vi "capex chambers.vi"(11 "stop":bool) -> ()   [LabVIEW 2013]
panel:
  in  "Minutes displayed":dbl=60.0
  out "Sensor 3 Temperature":waveform(dbl)(graph)={"t0"=timestamp(3552338969.221673 s since 1904-01-01), "dt"=0.001, "Y"=[19.008294294897723], "attributes"=variant("NI_ChannelName"=variant(string "Temp3"), "NI_UnitDescription"=variant(string "Amps"))}
  out "Sensor 3 Humidity":waveform(dbl)(graph)={"t0"=timestamp(3552338969.221658 s since 1904-01-01), "dt"=0.001, "Y"=[61.16415083954544], "attributes"=variant("NI_ChannelName"=variant(string "Humidity3"), "NI_UnitDescription"=variant(string "Amps"))}
  out "Sensor 2 Temperature":waveform(dbl)(graph)={"t0"=timestamp(3552338969.221643 s since 1904-01-01), "dt"=0.001, "Y"=[17.601047768518942], "attributes"=variant("NI_ChannelName"=variant(string "Temp2"), "NI_UnitDescription"=variant(string "Amps"))}
  out "Sensor 2 Humidity":waveform(dbl)(graph)={"t0"=timestamp(3552338969.221613 s since 1904-01-01), "dt"=0.001, "Y"=[70.37875059333966], "attributes"=variant("NI_ChannelName"=variant(string "Humidity2"), "NI_UnitDescription"=variant(string "Amps"))}
  out "Sensor 1 Temperature":waveform(dbl)(graph)={"t0"=timestamp(3552338969.221628 s since 1904-01-01), "dt"=0.001, "Y"=[17.486537818762628], "attributes"=variant("NI_ChannelName"=variant(string "Temp1"), "NI_UnitDescription"=variant(string "Amps"))}
  out "Sensor 1 Humidity":waveform(dbl)(graph)={"t0"=timestamp(3552338969.221598 s since 1904-01-01), "dt"=0.001, "Y"=[66.037122005], "attributes"=variant("NI_ChannelName"=variant(string "Humidity1"), "NI_UnitDescription"=variant(string "Amps"))}
  # "Chamber Temperatures and Humidities as reported by Omega boxes on walls"
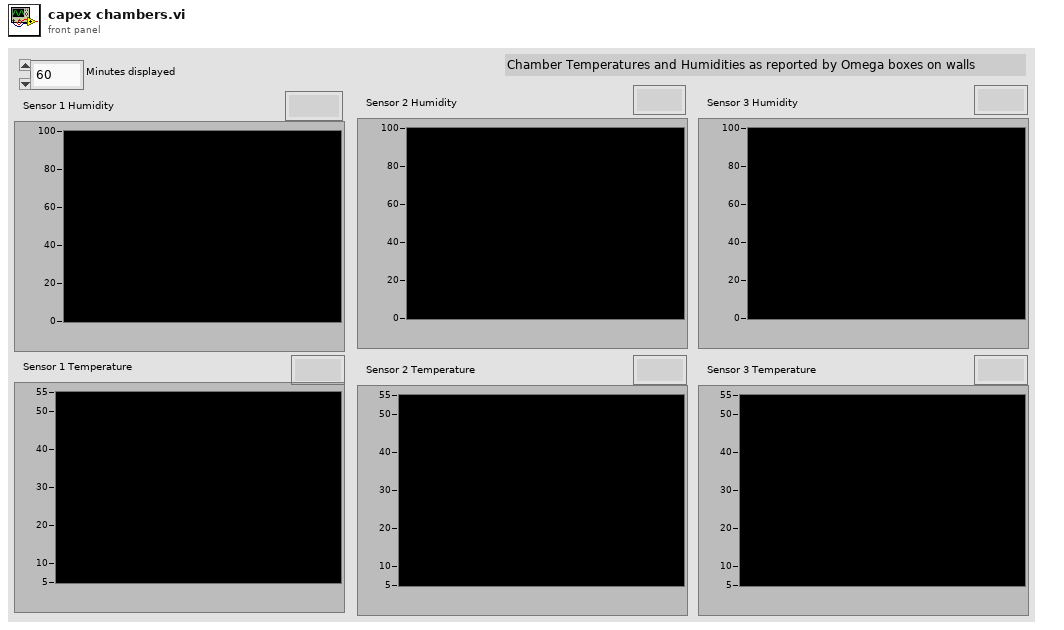
[diagram p1: front panel]
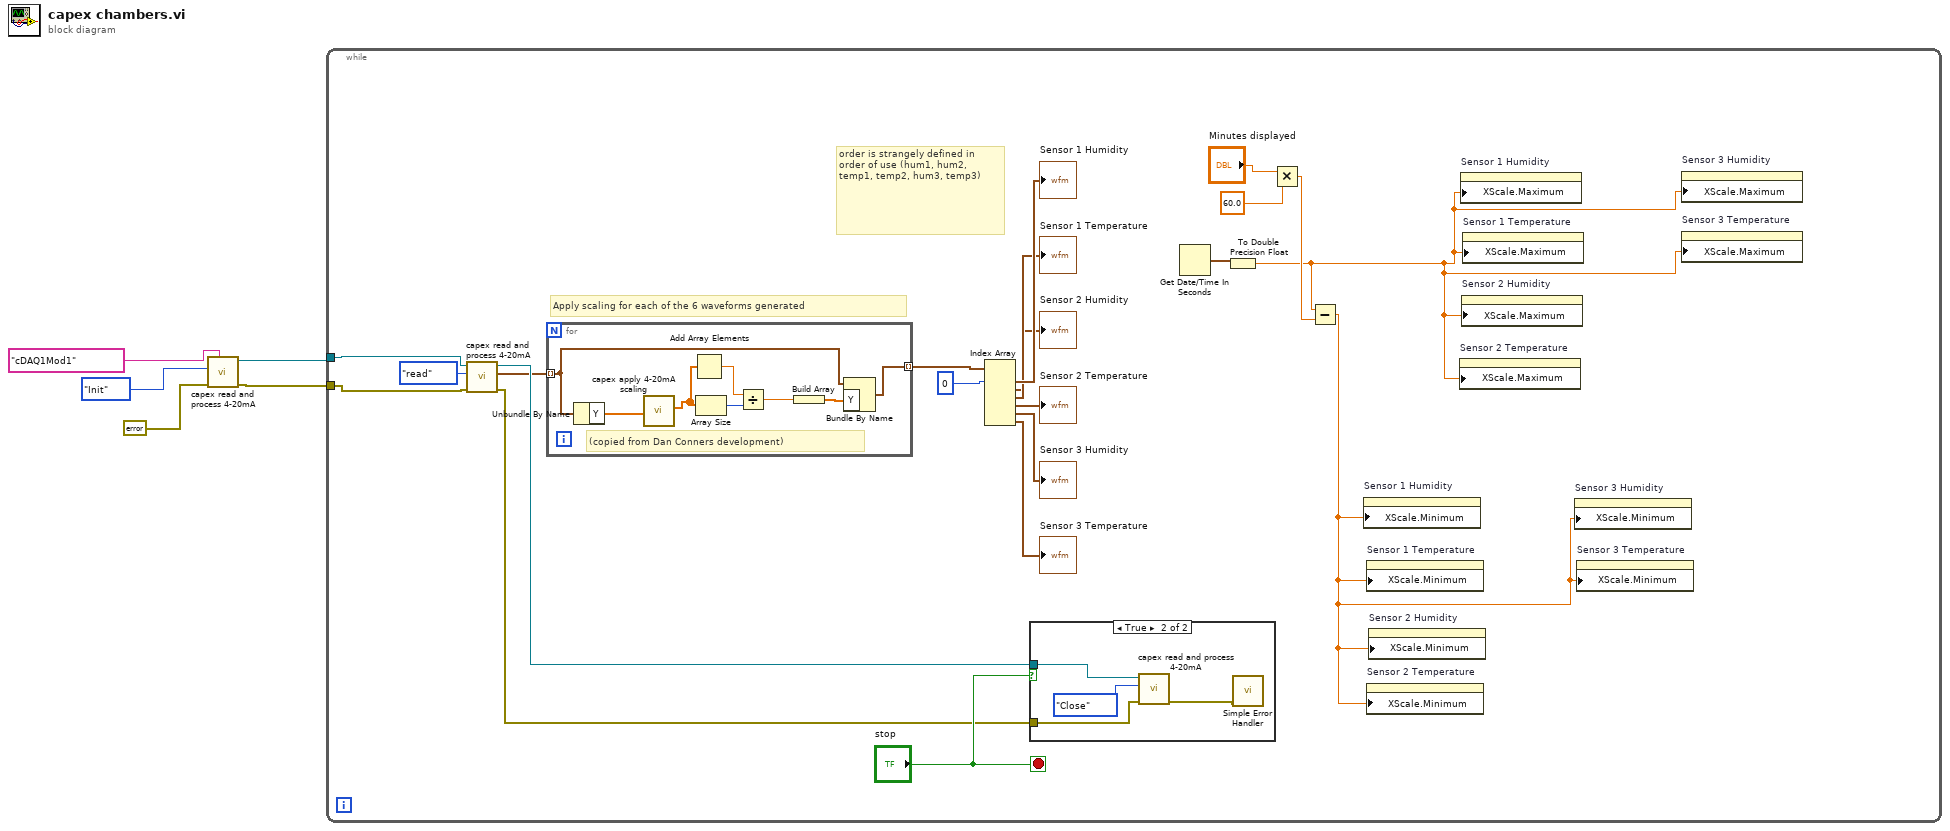
[diagram p0: block diagram]
diagram:
  n1 = call "capex read and process 4-20mA.vi"("DAQmx Device Name"=tag "cDAQ1Mod1", "error in"=errorcluster {"status"=FALSE, "code"=0, "source"=""}, "Command"=enum16{"Init", "read", "Close"}."Init") -> ("error out"=w1:errorcluster, "task out"=w3:refnum<k21>)  [unwired: 6 in, 1 out]
  n2 = while {
    tunnel: w3 -> [w10]
    tunnel: w1 -> [w9]
    stop <- "stop" stop-if-true
    # "Apply scaling for each of the 6 waveforms generated"
    # "order is strangely defined in order of use (hum1, hum2, temp1, temp2, hum3, temp3)"
    n3 = call "capex read and process 4-20mA.vi"("error in"=w9, "Command"=enum16{"Init", "read", "Close"}."read", "task in"=w10) -> ("error out"=w6:errorcluster, "data"=w8:waveform(dbl)[], "task out"=w12:refnum<k21>)  [unwired: 6 in]
    n4 = for {
      tunnel: w8 -> [w30] mode=indexing
      tunnel: [w29] -> w7 mode=indexing
      # "(copied from Dan Conners development)"
      n5 = Unbundle By Name(w30) -> ("Y"=w28:dbl[])
      n6 = call "capex apply 4-20mA scaling.vi"("Uncorrected Input"=w28) -> ("Corrected Array"=w27:dbl[])  [unwired: 8 in, 1 out]
      n7 = Add Array Elements(numeric array=w27) -> (sum=w32:dbl)
      n8 = Array Size(array=w27) -> (size(s)=w33:i32)
      n9 = Divide(x=w32, y=w33) -> (x/y=w34:dbl)
      n10 = Build Array(w34) -> (w31:dbl[])
      n11 = Bundle By Name(cluster=w30, "Y"=w31) -> (w29:waveform(dbl))
    }
    n12 = Index Array(array=w7, index #1=0 ("index")) -> (element #1=→"Sensor 1 Humidity":waveform(dbl), element #2=→"Sensor 2 Humidity":waveform(dbl), element #3=→"Sensor 1 Temperature":waveform(dbl), element #4=→"Sensor 2 Temperature":waveform(dbl), element #5=→"Sensor 3 Humidity":waveform(dbl), element #6=→"Sensor 3 Temperature":waveform(dbl))  [unwired: 5 in]
    n13 = case shown="True" "stop" {
      tunnel: w12 -> [_ w38]
      tunnel: w6 -> [_ w36]
      frame False {
      }
      frame True {
        n14 = call "capex read and process 4-20mA.vi"("error in"=w36, "Command"=enum16{"Init", "read", "Close"}."Close", "task in"=w38) -> ("error out"=w35:errorcluster)  [unwired: 6 in, 2 out]
        n15 = call <vilib>:"Simple Error Handler.vi"("error in (no error)"=w35) -> ()  [unwired: 4 in, 5 out]
      }
    }
    n16 = Get Date/Time In Seconds() -> (seconds since 1Jan1904=w16:timestamp)
    n17 = To Double Precision Float(number=w16) -> (double precision float=w14:dbl)
    n18 = Multiply(x="Minutes displayed", y=60.0) -> (x*y=w17:dbl)
    n19 = Subtract(x=w14, y=w17) -> (x-y=w15:dbl)
    n20 = property on="Sensor 1 Humidity" class="WFChart (strict)"("XScale.Minimum"=w15) -> ()  [unwired: 2 in, 2 out]
    n21 = property on="Sensor 1 Temperature" class="WFChart (strict)"("XScale.Minimum"=w15) -> ()  [unwired: 2 in, 2 out]
    n22 = property on="Sensor 2 Temperature" class="WFChart (strict)"("XScale.Minimum"=w15) -> ()  [unwired: 2 in, 2 out]
    n23 = property on="Sensor 2 Humidity" class="WFChart (strict)"("XScale.Minimum"=w15) -> ()  [unwired: 2 in, 2 out]
    n24 = property on="Sensor 2 Temperature" class="WFChart (strict)"("XScale.Maximum"=w14) -> ()  [unwired: 2 in, 2 out]
    n25 = property on="Sensor 1 Humidity" class="WFChart (strict)"("XScale.Maximum"=w14) -> ()  [unwired: 2 in, 2 out]
    n26 = property on="Sensor 2 Humidity" class="WFChart (strict)"("XScale.Maximum"=w14) -> ()  [unwired: 2 in, 2 out]
    n27 = property on="Sensor 1 Temperature" class="WFChart (strict)"("XScale.Maximum"=w14) -> ()  [unwired: 2 in, 2 out]
    n28 = property on="Sensor 3 Humidity" class="WFChart (strict)"("XScale.Minimum"=w15) -> ()  [unwired: 2 in, 2 out]
    n29 = property on="Sensor 3 Temperature" class="WFChart (strict)"("XScale.Minimum"=w15) -> ()  [unwired: 2 in, 2 out]
    n30 = property on="Sensor 3 Humidity" class="WFChart (strict)"("XScale.Maximum"=w14) -> ()  [unwired: 2 in, 2 out]
    n31 = property on="Sensor 3 Temperature" class="WFChart (strict)"("XScale.Maximum"=w14) -> ()  [unwired: 2 in, 2 out]
  }
